vi "Close Comm.vi"   [LabVIEW 2010]
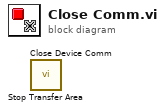
[diagram p0: block diagram]
diagram:
  n1 = call "Stop Transfer Area.vi"() -> ()  [unwired: 14 in, 2 out]
  n2 = call "Close Device Comm.vi"() -> ()  [unwired: 14 in, 2 out]
